vi "Untitled 3.vi"() -> ()   [LabVIEW 2016, in "Lutron QS Control Protocol.lvlib" / "Lutron QS Object.lvclass"]
uses:
  Lutron QS Object.lvclass
  Controls/Control System Visa Address and String cluster.ctl
  <vilib>/Instr/_visa.llb/VISA Find Search Mode.ctl
panel:
  out "Array 3":T1[](array[typedef])
  out "find list":string[](array[string])
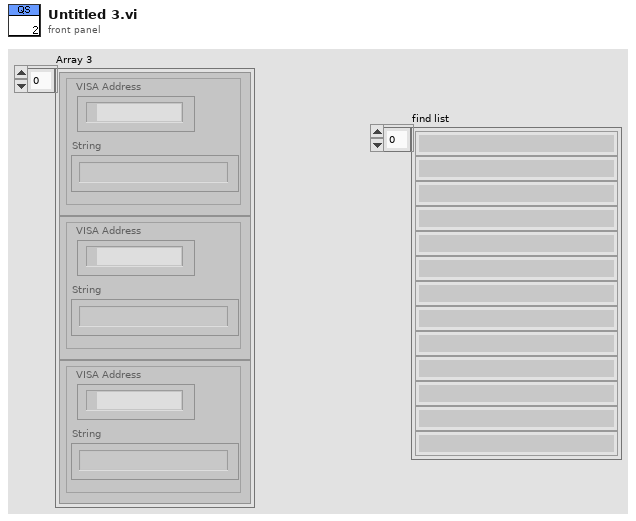
[diagram p1: front panel]
types:
  T1 = typedef "Control System Visa Address and String cluster.ctl" = cluster{"VISA Address":refnum<visa-resource-name>, "String":string}
  T2 = typedef "VISA Find Search Mode.ctl" = u32
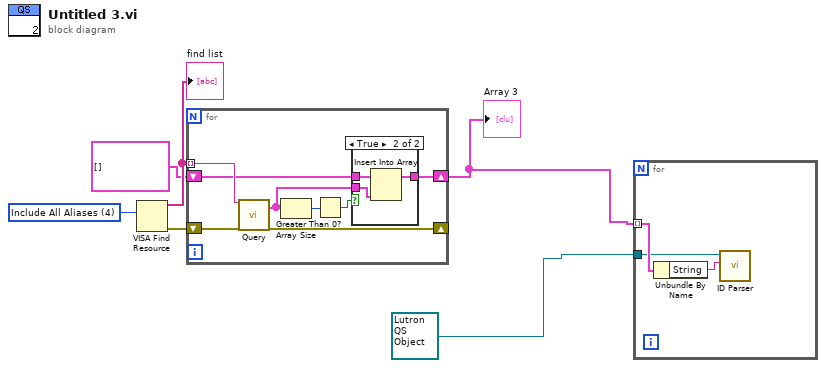
[diagram p0: block diagram]
diagram:
  w5 = T2 4 items=["Canonical Names Only"=0, "Aliases Only"=2, "Include Matching Aliases"=3, "Include All Aliases"=4] ("Search Mode")
  n1 = VISA Find Resource(10:w5) -> (0:w4:errorcluster, 3:w6:string[])  [unwired: 2 in, 1 out]
  "find list" <- w6
  n2 = for {
    tunnel: w6 -> [w14] mode=indexing
    shift-right: [w12] -> _
    shift-left: w4 -> [w13]
    shift-right: [w8] -> w2
    shift-left: T1[] [] ("Array 3") -> [w9]
    n3 = call "Query.vi"("VISA resource name"=w14, "error in (no error)"=w13) -> ("Array 3"=w7:T1[], "error out"=w12:errorcluster)  [unwired: 16 in]
    n4 = Array Size(array=w7) -> (size(s)=w11:i32)
    n5 = Greater Than 0?(x=w11) -> (x > 0?=w10:bool)
    n6 = case shown="True" w10 {
      tunnel: w9 -> [w15 w18]
      tunnel: [w15 w16] -> w8
      tunnel: w7 -> [_ w17]
      frame False {
      }
      frame True {
        n7 = Insert Into Array(array=w18, new element=w17) -> (w16:T1[])  [unwired: 1 in]
      }
    }
  }
  "Array 3" <- w2
  n8 = for {
    tunnel: w2 -> [w21] mode=indexing
    tunnel: refnum<class "Lutron QS Object.lvclass"> refnum ("Lutron QS Control Protocol.lvlib:Lutron QS Object.lvclass") -> [w19]
    n9 = Unbundle By Name(w21) -> ("String"=w20:string)
    n10 = call-dynamic "ID Parser.vi"("ID"=w20, "Lutron QS Object in"=w19) -> ()  [unwired: 8 in, 2 out]
  }
